vi "Dispense.vi"(8 "error in (no error)":errorcluster, 11 "Dispenser In":refnum<visa-resource-name>) -> (0 "error out":errorcluster, 3 "Dispenser Out":refnum<visa-resource-name>)   [LabVIEW 2018, in "Dispenser.lvclass"]
uses:
  Dispenser.lvclass
  Drivers/EFD Ultimus V/EFD Ultimus V.lvlib
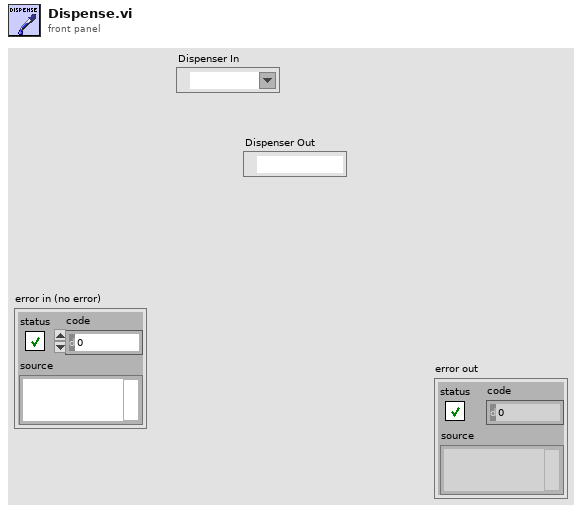
[diagram p1: front panel]
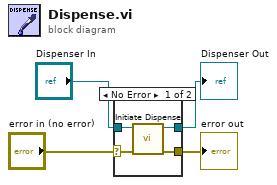
[diagram p0: block diagram]
diagram:
  n1 = case shown="No Error" "error in (no error)" {
    selector: "error in (no error)" -> [w6 w10]
    tunnel: [w5 w10] -> w3
    tunnel: "Dispenser In" -> [w8 w9]
    tunnel: [w7 w9] -> w1
    frame No Error {
      n2 = call "Initiate Dispense.vi"("error in (no error)"=w6, "VISA resource name"=w8) -> ("error out"=w5:errorcluster, "VISA resource name out"=w7:refnum<visa-resource-name>)  [unwired: 8 in]
    }
    frame Error {
    }
  }
  "error out" <- w3
  "Dispenser Out" <- w1
